vi "Basic Operations.vi"   [LabVIEW 2024, in "Libreria de reuso.lvlib"]
uses:
  Libreria de reuso.lvlib
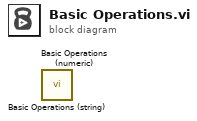
[diagram p0: block diagram]
diagram:
  n1 = call "Basic Operations (string).vi"() -> ()  [unwired: 11 in, 1 out]
  n2 = call "Basic Operations (numeric).vi"() -> ()  [unwired: 11 in, 1 out]
